vi "Version to HEX.vi"() -> ()   [LabVIEW 2015]
panel:
  in  "String":string="1.2.0.62"
  out "*(type *) &x 3":string
  out "*(type *) &x 2":string
  out "*(type *) &x":i64 format="%.0x"
  out "hex integer string":string
  in  "Version":i64=3288624
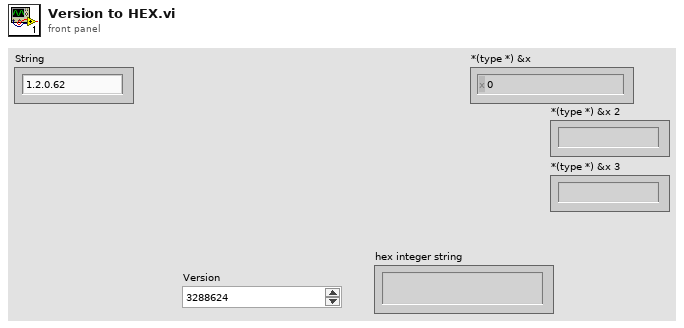
[diagram p1: front panel]
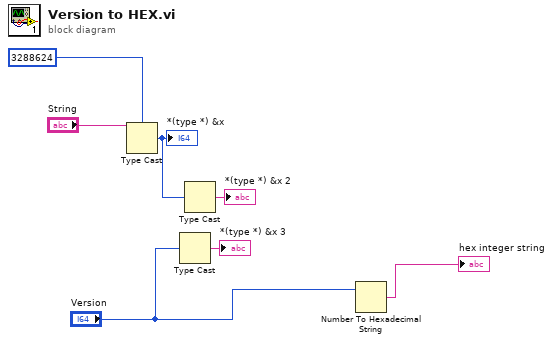
[diagram p0: block diagram]
diagram:
  n1 = Type Cast(type=i64 3288624 ("Version"), x="String") -> (*(type *) &x=w4:i64)
  "*(type *) &x" <- w4
  n2 = Type Cast(x="Version") -> (*(type *) &x=→"*(type *) &x 3":string)  [unwired: 1 in]
  n3 = Type Cast(x=w4) -> (*(type *) &x=→"*(type *) &x 2":string)  [unwired: 1 in]
  n4 = Number To Hexadecimal String(2:"Version") -> (0:→"hex integer string":string)  [unwired: 1 in]
